vi "click here.vi"() -> ()   [LabVIEW 2015]
uses:
  <vilib>/Utility/miscctls.llb/LVPositionTypeDef.ctl
panel:
  in  "stop":bool
  in  "Boolean":bool
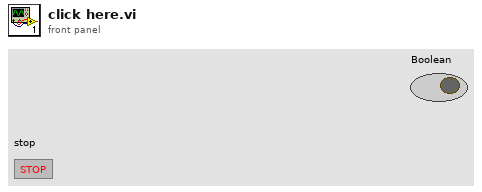
[diagram p1: front panel]
types:
  T1 = typedef "LVPositionTypeDef.ctl" = cluster{"Left":i32, "Top":i32}
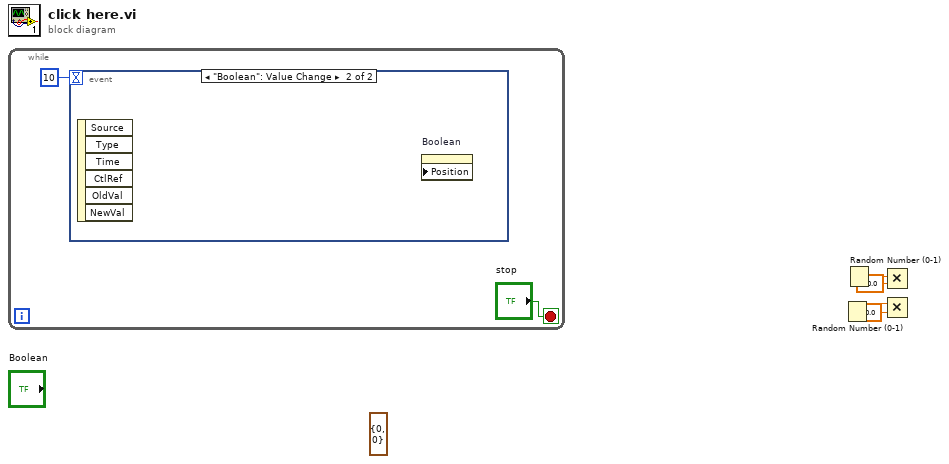
[diagram p0: block diagram]
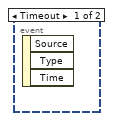
[diagram p2: hidden frame]
diagram:
  (unwired) T1 {"Left"=0, "Top"=0} ("Position")
  n1 = while {
    stop <- "stop" stop-if-true
    n2 = event shown="[1] \"Boolean\": Value Change" {
      selector: _ -> [_ _]
      dyn-events: _ -> [_ _]
      timeout: 10 -> [_ _]
      event Timeout {
        n3 = event-data() -> ()  [unwired: 1 in, 3 out]
      }
      event "Boolean": Value Change {
        n4 = event-data() -> ()  [unwired: 1 in, 6 out]
        n5 = property on="Boolean" class="Bool (strict)" props=["Position"]() -> ()  [unwired: 3 in, 2 out]
      }
    }
  }
  n6 = Random Number (0-1)() -> (number: 0 to 1=w3:dbl)
  n7 = Random Number (0-1)() -> (number: 0 to 1=w1:dbl)
  n8 = Multiply(x=w1, y=100.0) -> ()  [unwired: 1 out]
  n9 = Multiply(x=w3, y=100.0) -> ()  [unwired: 1 out]
